vi "Read Events Registrants.vi"(8 "Error In":errorcluster, 11 "Event Source In":refnum<class "Event Source Actor.lvclass">) -> (0 "Error Out":errorcluster, 1 "Registration Map":T1(c390), 3 "Event Source Out":refnum<class "Event Source Actor.lvclass">)   [LabVIEW 2021, in "EventSourceActor.lvlib" / "Event Source.lvlib" / "Event Source Actor.lvclass"]
doc: "This method returns a map of all subscriptions and can be used to understand more about which actors are subscribed for which events."
uses:
  Event Source Actor.lvclass
  Event Source Actor.lvclass/Event Source Actor.ctl
  <vilib>/ActorFramework/Message Enqueuer/Message Enqueuer.lvclass
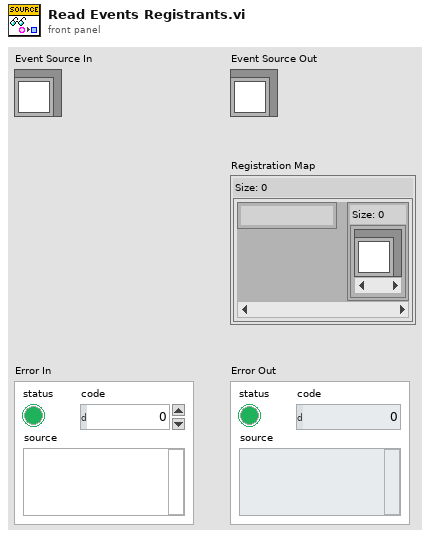
[diagram p1: front panel]
types:
  T1 = map{string, set{refnum<class "Message Enqueuer.lvclass">}}
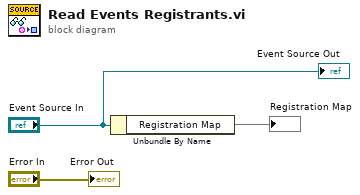
[diagram p0: block diagram]
diagram:
  n1 = Unbundle By Name("Event Source In") -> ("Registration Map"=→"Registration Map":T1)
  "Event Source Out" <- "Event Source In"
  "Error Out" <- "Error In"
